vi "4-wire-pre-logic.vi"(9 "ready for input in":bool, 10 "Input Valid in":bool, 11 "needs more iter in":bool) -> (1 "register state out":bool, 2 "excecute":bool, 3 "buffer input!":bool)   [LabVIEW 2018, in "SCTL.lvlib"]
uses:
  SCTL.lvlib
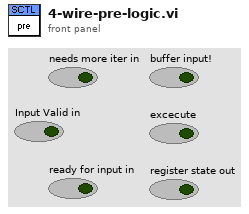
[diagram p1: front panel]
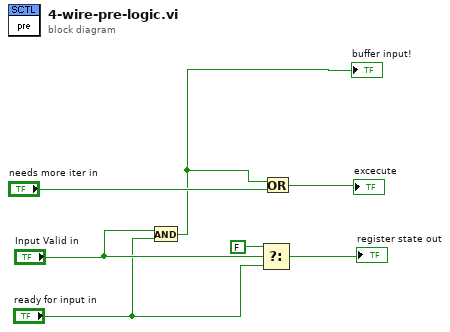
[diagram p0: block diagram]
diagram:
  n1 = And(x="Input Valid in", y="ready for input in") -> (x .and. y?=w1:bool)
  "buffer input!" <- w1
  n2 = Select(t=FALSE, s="Input Valid in", f="ready for input in") -> (s? t:f=→"register state out":bool)
  n3 = Or(x=w1, y="needs more iter in") -> (x .or. y?=→"excecute":bool)
